vi "knownhosts_delete.vi"() -> ()   [LabVIEW 2013]
doc: "Illustrates how to delete a host key from a host key database."
uses:
  libssh2/libssh2_knownhost.ctl
  libssh2/Host Key Refnum.ctl
  libssh2/libssh2_init_default.vi
  libssh2/libssh2.lvlib
panel:
  out "error out":errorcluster
  out "known hosts":T1[](array[typedef])
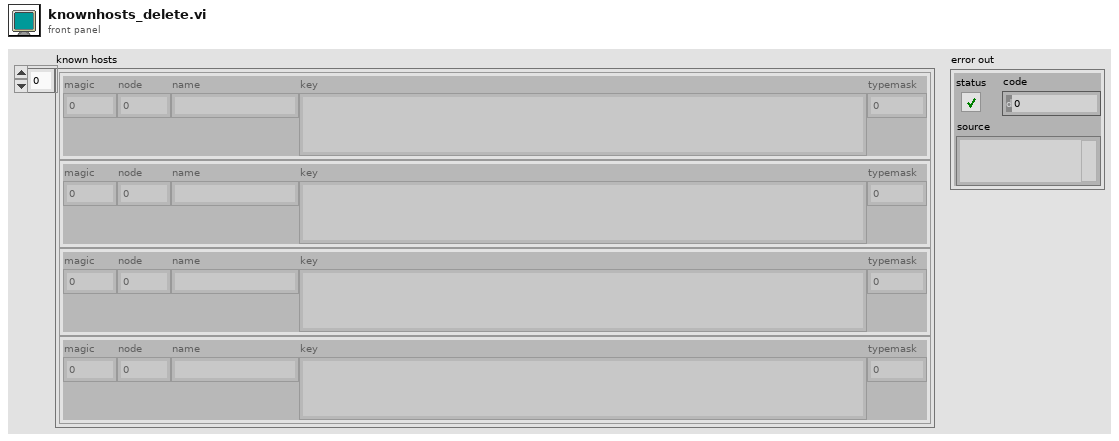
[diagram p1: front panel]
types:
  T1 = typedef "libssh2.lvlib/libssh2_knownhost.ctl" = cluster{"magic":u32, "node":u64, "name":string, "key":string, "typemask":i32}
  T2 = typedef "libssh2.lvlib/Host Key Refnum.ctl" = refnum<k1>
  T3 = typedef "libssh2.lvlib/Session Refnum.ctl" = refnum<k1>
  T4 = typedef "libssh2.lvlib/Host Key Database Refnum.ctl" = refnum<k1>
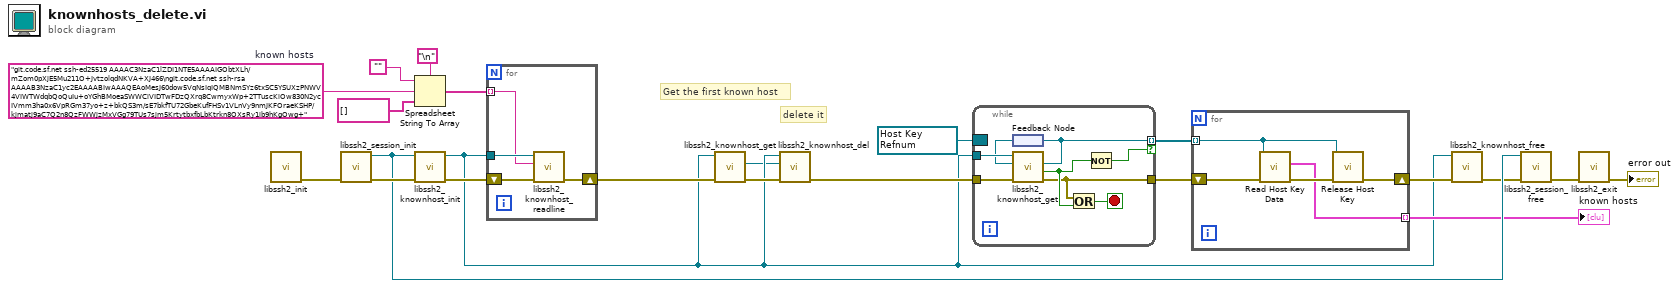
[diagram p0: block diagram]
diagram:
  w12 = "git.code.sf.net ssh-ed25519 AAAAC3NzaC1lZDI1NTE5AAAAIGObtXLh/mZom0pXjE5Mu211O+JvtzolqdNKVA+XJ466\ngit.code.sf.net ssh-rsa AAAAB3NzaC1yc2EAAAABIwAAAQEAoMesJ60dow5VqNsIqIQMBNmSYz6txSC5YSUXzPNWV4VIWTWdqbQoQuIu+oYGhBMoeaSWWCiVIDTwFDzQXrq8CwmyxWp+2TTuscKiOw830N2ycIVmm3ha0x6VpRGm37yo+z+bkQS3m/sE7bkfTU72GbeKufFHSv1VLnVy9nmJKFOraeKSHP/kjmatj9aC7Q2n8QzFWWjzMxVGg79TUs7sjm5KrtytbxfbLbKtrkn8OXsRy1ib9hKgOwg+"  # known hosts
  w14 = T2 refnum items=["host key"] ("next")
  # "delete it"
  # "Get the first known host"
  n1 = call-poly "libssh2_init.vi"() -> ("error out"=w22:errorcluster)  [unwired: 11 in]
  n2 = call "libssh2_session_init.vi"("error in (no error)"=w22) -> ("error out"=w21:errorcluster, "session"=w20:T3)  [unwired: 9 in]
  n3 = Spreadsheet String To Array(delimiter (Tab)="\n", format string="", spreadsheet string=w12, array type (2D Dbl)=string[] []) -> (array=w11:string[])
  n4 = call "libssh2_knownhost_init.vi"("error in (no error)"=w21, "session"=w20) -> ("error out"=w17:errorcluster, "host key database"=w2:T4)  [unwired: 8 in]
  n5 = for {
    tunnel: w2 -> [w24]
    tunnel: w11 -> [w23] mode=indexing
    shift-right: [w25] -> w5
    shift-left: w17 -> [w26]
    n6 = call "libssh2_knownhost_readline.vi"("error in (no error)"=w26, "line"=w23, "host key database"=w24) -> ("error out"=w25:errorcluster)  [unwired: 8 in]
  }
  n7 = call "libssh2_knownhost_get.vi"("error in (no error)"=w5, "host key database"=w2) -> ("error out"=w4:errorcluster, "host key"=w1:T2)  [unwired: 7 in, 1 out]
  n8 = call "libssh2_knownhost_del.vi"("error in (no error)"=w4, "host key"=w1, "host key database"=w2) -> ("error out"=w3:errorcluster)  [unwired: 8 in]
  n9 = while {
    tunnel: w3 -> [w34]
    tunnel: [w28] -> w16
    tunnel: w2 -> [w33]
    border: w14 -> [_]
    tunnel: [w30] -> w13 mode=indexing if=w27
    stop <- w32 stop-if-true
    n10 = feedback #1() -> (w31:T2)
    n11 = call "libssh2_knownhost_get.vi"("error in (no error)"=w34, "previous host key"=w31, "host key database"=w33) -> ("error out"=w28:errorcluster, "end reached"=w29:bool, "host key"=w30:T2)  [unwired: 6 in]
    n12 = feedback-in #1(w30) -> ()
    n13 = Or(x=w28, y=w29) -> (x .or. y?=w32:bool)
    n14 = Not(x=w29) -> (.not. x?=w27:bool)
  }
  n15 = for {
    shift-right: [w39] -> w15
    shift-left: w16 -> [w38]
    tunnel: w13 -> [w35] mode=indexing
    tunnel: [w36] -> w7 mode=indexing
    n16 = call "Read Host Key Data.vi"("error in (no error)"=w38, "host key"=w35) -> ("error out"=w37:errorcluster, "host key data"=w36:T1)  [unwired: 8 in]
    n17 = call "Release Host Key.vi"("error in (no error)"=w37, "host key"=w35) -> ("error out"=w39:errorcluster)  [unwired: 9 in]
  }
  "known hosts" <- w7
  n18 = call "libssh2_knownhost_free.vi"("error in (no error)"=w15, "host key database"=w2) -> ("error out"=w19:errorcluster)  [unwired: 9 in]
  n19 = call "libssh2_session_free.vi"("error in (no error)"=w19, "session"=w20) -> ("error out"=w18:errorcluster)  [unwired: 9 in]
  n20 = call "libssh2_exit.vi"("error in (no error)"=w18) -> ("error out"=→"error out":errorcluster)  [unwired: 10 in]
